vi "DHE_FormatNightID.vi"(10 "IDbase in":string) -> (2 "expID out":string)   [LabVIEW 2016]
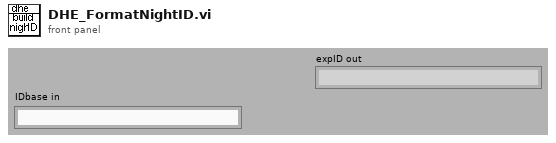
[diagram p1: front panel]
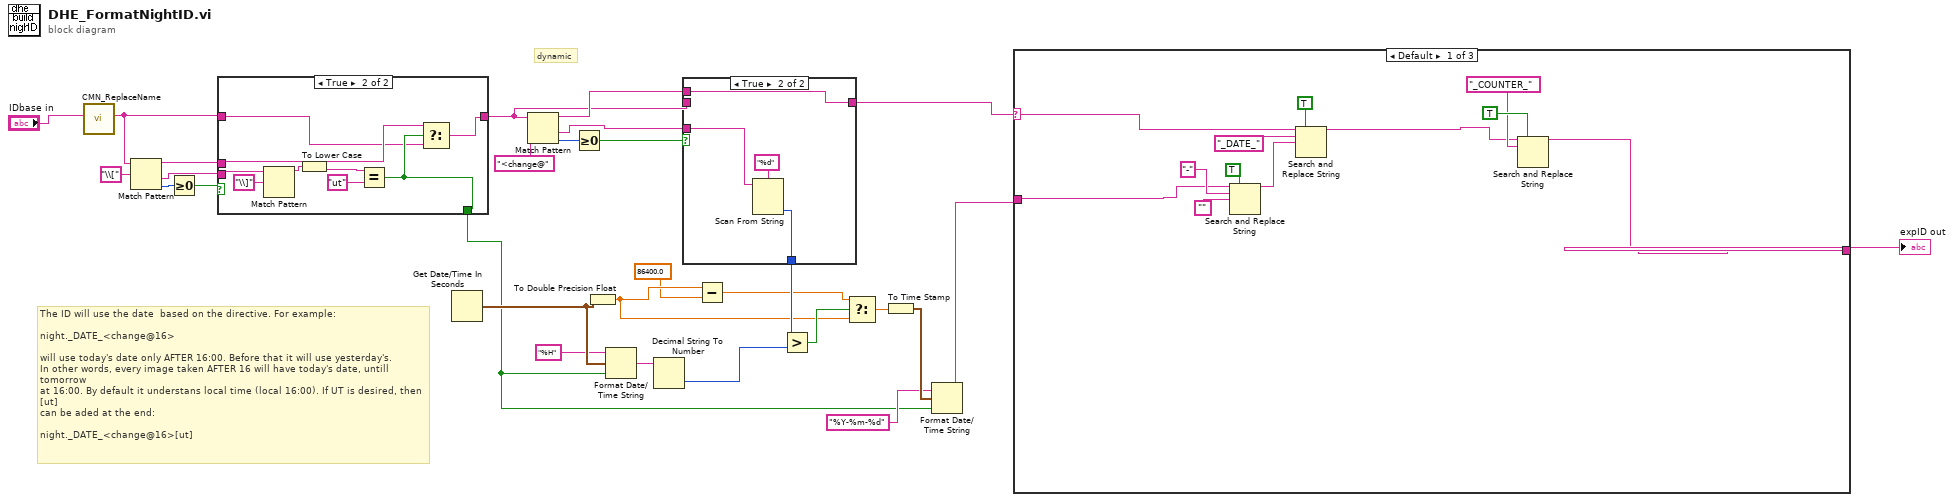
[diagram p0: block diagram]
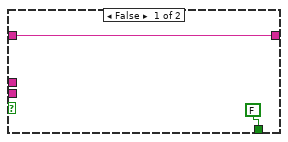
[diagram p2: hidden frame]
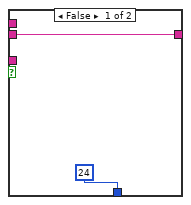
[diagram p3: hidden frame]
diagram:
  # "The ID will use the date  based on the directive. For example:\n\nnight._DATE_<change@16>\n\nwill use today's date only AFTER 16:00. Before that it will use yesterday's.\nIn other words, every image taken AFTER 16 will have today's date, untill tomorrow\nat 16:00. By default it understans local time (local 16:00). If UT is desired, then [ut] \ncan be aded at the end:\n\nnight._DATE_<change@16>[ut]"
  # "dynamic"
  n1 = call "CMN_ReplaceName.vi"("name in"="IDbase in") -> ("name out"=w7:string)  [unwired: 1 in, 9 out]
  n2 = Match Pattern(string=w7, regular expression="\\[") -> (before substring=w5:string, after substring=w4:string, offset past match=w9:i32)  [unwired: 2 out]
  n3 = Greater Or Equal To 0?(x=w9) -> (x >= 0?=w8:bool)
  n4 = case shown="True" w8 {
    tunnel: w7 -> [w31 w33]
    tunnel: [w31 w32] -> w6
    tunnel: w5 -> [_ w34]
    tunnel: w4 -> [_ w39]
    tunnel: [FALSE w35] -> w3
    frame False {
    }
    frame True {
      n5 = Match Pattern(string=w39, regular expression="\\]") -> (before substring=w37:string)  [unwired: 4 out]
      n6 = To Lower Case(string=w37) -> (all lower case string=w36:string)
      n7 = Equal?(x=w36, y="ut") -> (x = y?=w35:bool)
      n8 = Select(t=w34, s=w35, f=w33) -> (s? t:f=w32:string)
    }
  }
  n9 = Get Date/Time In Seconds() -> (seconds since 1Jan1904=w27:timestamp)
  n10 = Match Pattern(string=w6, regular expression="<change@") -> (before substring=w13:string, after substring=w21:string, offset past match=w23:i32)  [unwired: 2 out]
  n11 = Greater Or Equal To 0?(x=w23) -> (x >= 0?=w22:bool)
  n12 = To Double Precision Float(number=w27) -> (double precision float=w2:dbl)
  n13 = Format Date/Time String(time format string (%c)="%H", seconds (now)=w27, UTC format=w3) -> (date/time string=w25:string)
  n14 = Decimal String To Number(string=w25) -> (number=w19:i32)  [unwired: 3 out]
  n15 = case shown="True" w22 {
    tunnel: w6 -> [w42 _]
    tunnel: [w42 w44] -> w12
    tunnel: w21 -> [_ w43]
    tunnel: [24 w46] -> w20
    tunnel: w13 -> [_ w44]
    frame False {
    }
    frame True {
      n16 = Scan From String(format string="%d", input string=w43) -> (output 1=w46:i32)  [unwired: 2 in, 4 out]
    }
  }
  n17 = Subtract(x=w2, y=86400.0 ("x")) -> (x-y=w17:dbl)
  n18 = Greater?(x=w20, y=w19) -> (0:w18:bool)
  n19 = Select(t=w17, s=w18, f=w2) -> (s? t:f=w16:dbl)
  n20 = To Time Stamp(1:w16) -> (0:w15:timestamp)
  n21 = Format Date/Time String(time format string (%c)="%Y-%m-%d", seconds (now)=w15, UTC format=w3) -> (date/time string=w14:string)
  n22 = case shown="Default" w12 {
    selector: w12 -> [w58 _ _]
    tunnel: w14 -> [w48 w59 w60]
    tunnel: [w47 w59 w60] -> w29
    frame Default {
      n23 = Search and Replace String(replace all?=TRUE ("replace all? (F)"), input string=w48, search string="-", replace string="") -> (result string=w52:string)  [unwired: 1 in, 6 out]
      n24 = Search and Replace String(replace all?=TRUE ("replace all? (F)"), input string=w58, search string="_DATE_", replace string=w52) -> (result string=w49:string)  [unwired: 1 in, 6 out]
      n25 = Search and Replace String(replace all?=TRUE ("replace all? (F)"), input string=w49, search string="_COUNTER_") -> (result string=w47:string)  [unwired: 1 in, 7 out]
    }
    frame "_UNDEF_" {
    }
    frame "_UT_" {
    }
  }
  "expID out" <- w29
